vi "measure_v.vi"(8 "error in (no error)":errorcluster, 10 "Channel":string="1", 11 "VISA Refnum in":refnum<visa-resource-name>) -> (0 "error out":errorcluster, 2 "V readback (V)":dbl, 3 "VISA Refnum out":refnum<visa-resource-name>)   [LabVIEW 2018]
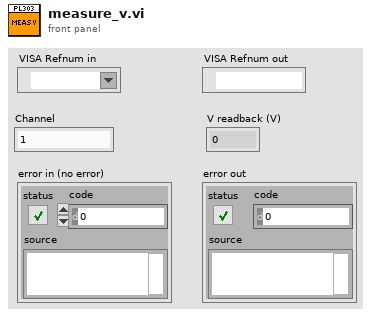
[diagram p1: front panel]
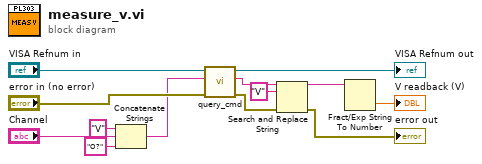
[diagram p0: block diagram]
diagram:
  n1 = Concatenate Strings("V" ("string"), "Channel", "O?" ("string")) -> (w6:string)
  n2 = call "query_cmd.vi"("error in (no error)"="error in (no error)", "write buffer"=w6, "VISA Refnum in"="VISA Refnum in") -> ("error out"=w3:errorcluster, "String"=w5:string, "VISA Refnum out"=→"VISA Refnum out":refnum<visa-resource-name>)  [unwired: 6 in]
  n3 = Search and Replace String(input string=w5, search string="V", error in=w3) -> (result string=w1:string, error out=→"error out":errorcluster)  [unwired: 5 in, 2 out]
  n4 = Fract/Exp String To Number(string=w1) -> (number=→"V readback (V)":dbl)  [unwired: 3 in, 1 out]
